vi "H_check_2.vi"(9 "Sweep\nTolerance %":dbl=0.1, 10 "H_in":dbl, 11 "H_target (K)":dbl) -> (3 "= H target":bool)   [LabVIEW 2016]
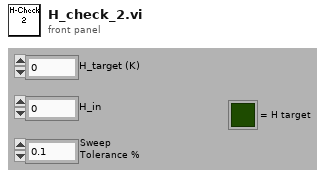
[diagram p1: front panel]
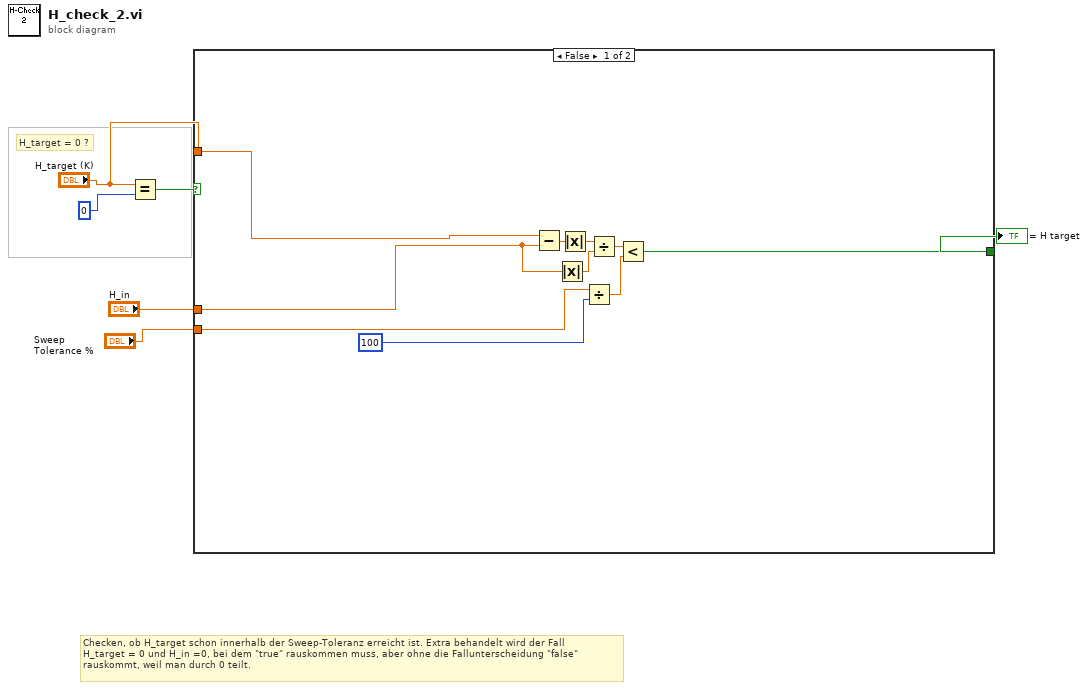
[diagram p0: block diagram]
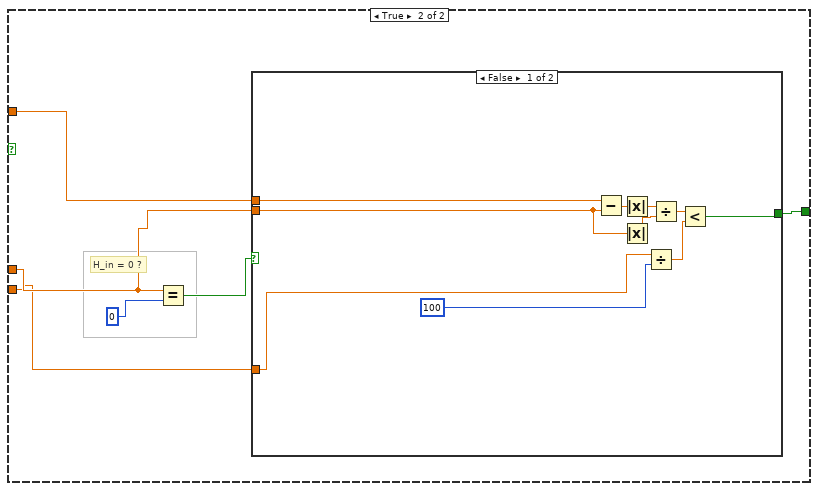
[diagram p2: hidden frame]
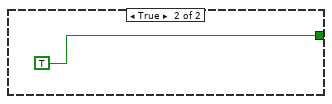
[diagram p3: hidden frame]
diagram:
  # "Checken, ob H_target schon innerhalb der Sweep-Toleranz erreicht ist. Extra behandelt wird der Fall\nH_target = 0 und H_in =0, bei dem \"true\" rauskommen muss, aber ohne die Fallunterscheidung \"false\"\nrauskommt, weil man durch 0 teilt."
  # "H_target = 0 ?"
  n1 = Equal?(x="H_target (K)", y=0) -> (x = y?=w5:bool)
  n2 = case shown="False" w5 {
    tunnel: "H_target (K)" -> [w11 w21]
    tunnel: [w10 w22] -> w3
    tunnel: "H_in" -> [w8 w19]
    tunnel: "Sweep\nTolerance %" -> [w9 w17]
    frame False {
      n3 = Subtract(x=w11, y=w8) -> (x-y=w12:dbl)
      n4 = Absolute Value(x=w8) -> (abs(x)=w7:dbl)
      n5 = Absolute Value(x=w12) -> (abs(x)=w13:dbl)
      n6 = Divide(x=w9, y=100) -> (x/y=w15:dbl)
      n7 = Divide(x=w13, y=w7) -> (x/y=w14:dbl)
      n8 = Less?(x=w14, y=w15) -> (x < y?=w10:bool)
    }
    frame True {
      # "H_in = 0 ?"
      n9 = Equal?(x=w19, y=0) -> (x = y?=w18:bool)
      n10 = case shown="False" w18 {
        tunnel: [w26 TRUE] -> w22
        tunnel: w21 -> [w27 _]
        tunnel: w19 -> [w24 _]
        tunnel: w17 -> [w25 _]
        frame False {
          n11 = Subtract(x=w27, y=w24) -> (x-y=w28:dbl)
          n12 = Absolute Value(x=w28) -> (abs(x)=w29:dbl)
          n13 = Absolute Value(x=w24) -> (abs(x)=w23:dbl)
          n14 = Divide(x=w25, y=100) -> (x/y=w31:dbl)
          n15 = Divide(x=w29, y=w23) -> (x/y=w30:dbl)
          n16 = Less?(x=w30, y=w31) -> (x < y?=w26:bool)
        }
        frame True {
        }
      }
    }
  }
  "= H target" <- w3
